vi "Verbosity Test.vi"(8 "error in (no error)":errorcluster) -> (0 "error out":errorcluster)   [LabVIEW 2013]
uses:
  classes/Assert/Assert True.vi
  classes/Assert/Assert False.vi
  classes/Assert/Assert Error.vi
  classes/Assert/Assert Not Error.vi
  classes/Assert/Assert Equal Value_Variant.vi
  classes/Assert/Assert Greater_Variant.vi
  classes/Assert/Assert Less Or Equal_Variant.vi
  classes/Test/Test.lvclass
  classes/Assert/Assert.lvclass
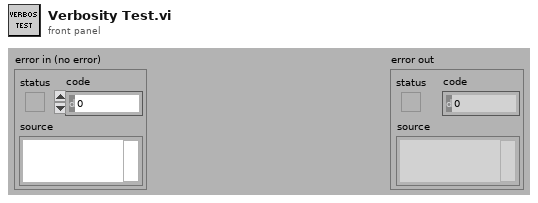
[diagram p1: front panel]
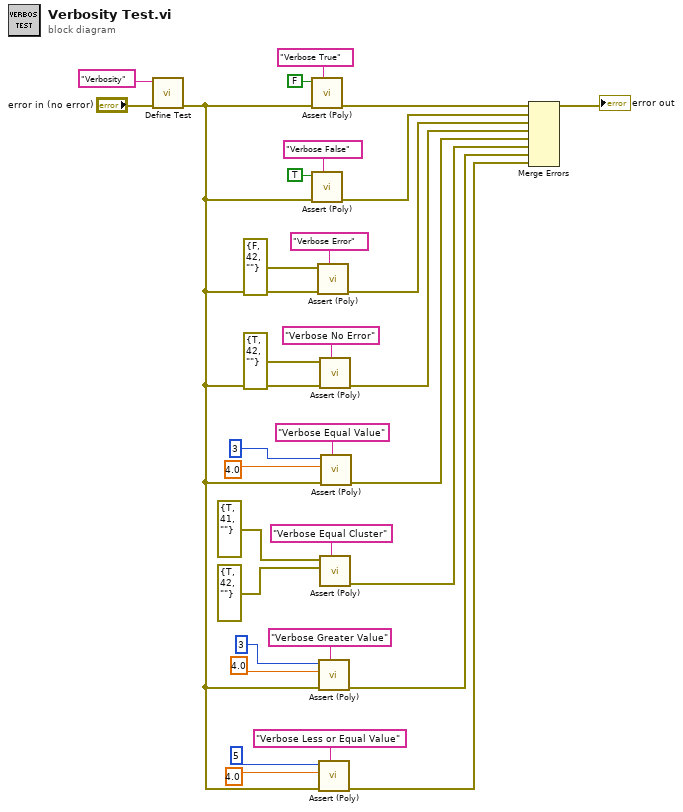
[diagram p0: block diagram]
diagram:
  n1 = call "Define Test.vi"("error in (no error)"="error in (no error)", "Label (VI Title)"="Verbosity" ("Label")) -> ("error out"=w11:errorcluster)  [unwired: 9 in]
  n2 = call-poly "Assert (Poly).vi"("Label"="Verbose True", "error in (no error)"=w11, "True?"=FALSE) -> ("error out"=w28:errorcluster)  [unwired: 8 in]
  n3 = call-poly "Assert (Poly).vi"("Label"="Verbose False", "error in (no error)"=w11, "False?"=TRUE) -> ("error out"=w24:errorcluster)  [unwired: 8 in]
  n4 = call-poly "Assert (Poly).vi"("Label"="Verbose Error", "error in (no error)"=w11, "Error?"=errorcluster {"status"=FALSE, "code"=42, "source"=""}) -> ("error out"=w22:errorcluster)  [unwired: 8 in]
  n5 = call-poly "Assert (Poly).vi"("Label"="Verbose Greater Value", "error in (no error)"=w11, "Y"=4.0, "X"=3) -> ("error out"=w13:errorcluster)  [unwired: 7 in]
  n6 = call-poly "Assert (Poly).vi"("Label"="Verbose Less or Equal Value", "error in (no error)"=w11, "Y"=4.0, "X"=5) -> ("error out"=w12:errorcluster)  [unwired: 7 in]
  n7 = call-poly "Assert (Poly).vi"("Label"="Verbose No Error", "error in (no error)"=w11, "Not Error?"=errorcluster {"status"=TRUE, "code"=42, "source"=""}) -> ("error out"=w18:errorcluster)  [unwired: 8 in]
  n8 = call-poly "Assert (Poly).vi"("Label"="Verbose Equal Cluster", "Y"=errorcluster {"status"=TRUE, "code"=42, "source"=""} ("Not Error?"), "X"=errorcluster {"status"=TRUE, "code"=41, "source"=""} ("Not Error?")) -> ("error out"=w1:errorcluster)  [unwired: 8 in]
  n9 = call-poly "Assert (Poly).vi"("Label"="Verbose Equal Value", "error in (no error)"=w11, "Y"=4.0, "X"=3) -> ("error out"=w14:errorcluster)  [unwired: 7 in]
  n10 = Merge Errors(w28, w24, w22, w18, w14, w1, w13, w12) -> (→"error out":errorcluster)
